vi "Dispense test - Copy.vi"() -> ()   [LabVIEW 2019]
uses:
  Classes/Controller/Dispenser/Dispenser.lvclass
  Classes/Controller/I-O/I-O.lvclass
  Classes/Controller/Controller.lvclass
panel:
  out "stop after dispensing":bool
  out "Value":bool
  out "error out":errorcluster
  in  "error in (no error)":errorcluster
  in  "Pressure":i16=20
  in  "Dispense":bool
  in  "stop":bool
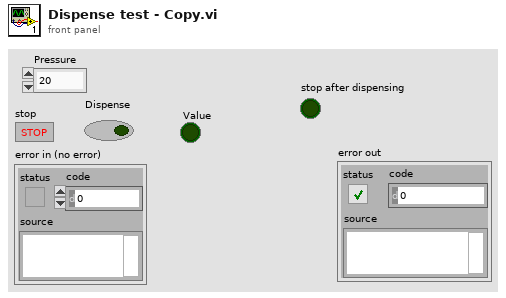
[diagram p1: front panel]
types:
  T1 = typedef "Controller.lvclass/Controllers.ctl" = cluster{"I-O.lvclass":refnum<class "I-O.lvclass">, "Dispenser.lvclass":refnum<class "Dispenser.lvclass">, "Gantry":refnum<k24>}
  T2 = typedef "I-O.lvclass/Pin Map.ctl" = cluster{"Region Valves":i32[], "Extra Valves":dbl[][][], "Tool Primary Valve":i32, "Tool Secondary Valve":i32, "Region Sensors":i32[], "Extra Sensors":dbl[][][], "Tool Primary Sensor":dbl, "Tool Secondary Sensor":dbl, "Compression Sensor":dbl, "5V":i32, "Dispener":dbl}
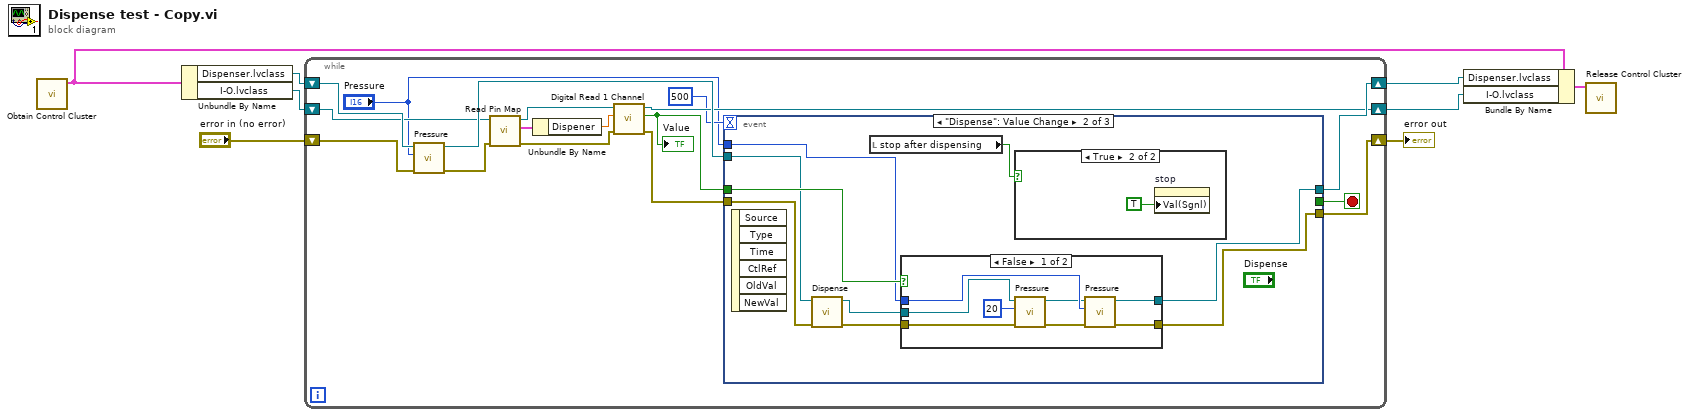
[diagram p0: block diagram]
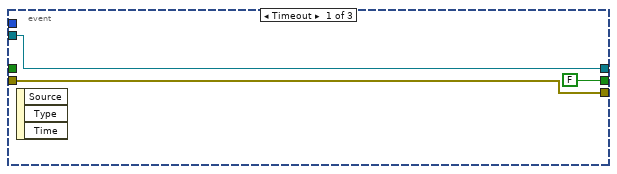
[diagram p2: hidden frame]
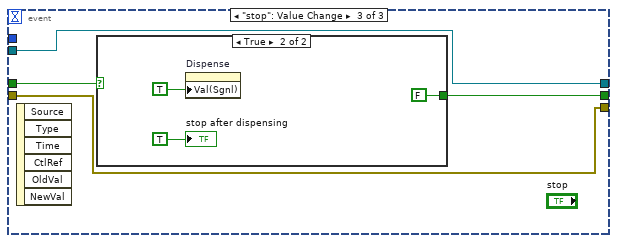
[diagram p5: hidden frame]
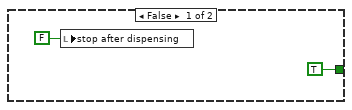
[diagram p6: hidden frame]
diagram:
  n1 = call "Obtain Control Cluster.vi"() -> ("Control Out"=w7:T1)  [unwired: 11 in]
  n2 = Unbundle By Name(w7) -> ("Dispenser.lvclass"=w3:refnum<class "Dispenser.lvclass">, "I-O.lvclass"=w2:refnum<class "I-O.lvclass">)
  n3 = while {
    shift-right: [w23] -> w5
    shift-left: w3 -> [w22]
    shift-right: [w24] -> w6
    shift-left: "error in (no error)" -> [w18]
    shift-right: [w11] -> w1
    shift-left: w2 -> [w19]
    stop <- w21 stop-if-true
    n4 = call-dynamic "Pressure.vi"("error in (no error)"=w18, "Pressure"="Pressure", "Dispenser in"=w22) -> ("error out"=w14:errorcluster, "Dispenser out"=w25:refnum<class "Dispenser.lvclass">)  [unwired: 7 in]
    n5 = call-dynamic "Read Pin Map.vi"("error in (no error)"=w14, "I-O in"=w19) -> ("error out"=w15:errorcluster, "Pin Map 2"=w20:T2, "I-O out"=w17:refnum<class "I-O.lvclass">)  [unwired: 7 in]
    n6 = Unbundle By Name(w20) -> ("Dispener"=w16:dbl)
    n7 = call-dynamic "Digital Read 1 Channel.vi"("error in (no error)"=w15, "Read"=w16, "I-O in"=w17) -> ("error out"=w13:errorcluster, "Value"=w12:bool, "I-O out"=w11:refnum<class "I-O.lvclass">)  [unwired: 6 in]
    "Value" <- w12
    n8 = event shown="[1] \"Dispense\": Value Change" {
      selector: _ -> [_ _ _]
      dyn-events: _ -> [_ _ _]
      timeout: 500 -> [_ _ _]
      tunnel: w25 -> [w26 w34 w49]
      tunnel: [w26 w30 w49] -> w23
      tunnel: w13 -> [w28 w33 w52]
      tunnel: [w28 w29 w52] -> w24
      tunnel: [FALSE ("stop after dispensing") _ w50] -> w21
      tunnel: w12 -> [_ w36 w51]
      tunnel: "Pressure" -> [_ w35 _]
      event Timeout {
        n9 = event-data() -> ()  [unwired: 1 in, 3 out]
      }
      event "Dispense": Value Change {
        n10 = event-data() -> ()  [unwired: 1 in, 6 out]
        n11 = call-dynamic "Dispense.vi"("error in (no error)"=w33, "Dispenser in"=w34) -> ("error out"=w31:errorcluster, "Dispenser out"=w32:refnum<class "Dispenser.lvclass">)  [unwired: 8 in]
        n12 = local read "stop after dispensing"() -> (w37:bool)
        n13 = case shown="False" w36 {
          tunnel: w32 -> [w45 w47]
          tunnel: [w40 w47] -> w30
          tunnel: w31 -> [w44 w46]
          tunnel: [w41 w46] -> w29
          tunnel: w35 -> [w42 _]
          frame False {
            n14 = call-dynamic "Pressure.vi"("error in (no error)"=w44, "Pressure"=i16 20, "Dispenser in"=w45) -> ("error out"=w43:errorcluster, "Dispenser out"=w38:refnum<class "Dispenser.lvclass">)  [unwired: 7 in]
            n15 = call-dynamic "Pressure.vi"("error in (no error)"=w43, "Pressure"=w42, "Dispenser in"=w38) -> ("error out"=w41:errorcluster, "Dispenser out"=w40:refnum<class "Dispenser.lvclass">)  [unwired: 7 in]
          }
          frame True {
          }
        }
        n16 = case shown="True" w37 {
          frame False {
          }
          frame True {
            n17 = property on="stop" class="Bool (strict)"("Val(Sgnl)"=TRUE ("Value (Signaling)")) -> ()  [unwired: 2 in, 2 out]
          }
        }
      }
      event "stop": Value Change {
        n18 = event-data() -> ()  [unwired: 1 in, 6 out]
        n19 = case shown="True" w51 {
          tunnel: [TRUE FALSE] -> w50
          frame False {
            n20 = local write "stop after dispensing"(FALSE ("stop after dispensing")) -> ()
          }
          frame True {
            n21 = property on="Dispense" class="Bool (strict)"("Val(Sgnl)"=TRUE ("Value (Signaling)")) -> ()  [unwired: 2 in, 2 out]
            "stop after dispensing" <- TRUE ("stop after dispensing")
          }
        }
      }
    }
  }
  "error out" <- w6
  n22 = Bundle By Name(cluster=w7, "Dispenser.lvclass"=w5, "I-O.lvclass"=w1) -> (w4:T1)
  n23 = call "Release Control Cluster.vi"("output cluster"=w4) -> ()  [unwired: 11 in]
